vi "demo_Comparison Reports from CLI.vi"(11 "Stop Demo":refnum<user-event>) -> ()   [LabVIEW 2020]
panel:
  # "LabVIEW 2025 Q3 Beta - Comparison Reports from LabVIEW CLI\n\nThe LabVIEW CLI now includes the CreateComparisonReport operation which will generate VI Comparison reports. You can specify a report type of HTML, HTML (Single File), Microsoft Word, Plain Text, or XML.\n\nLearn more about the LabVIEW 2025 Q3 Beta program at https://www.ni.com/beta."
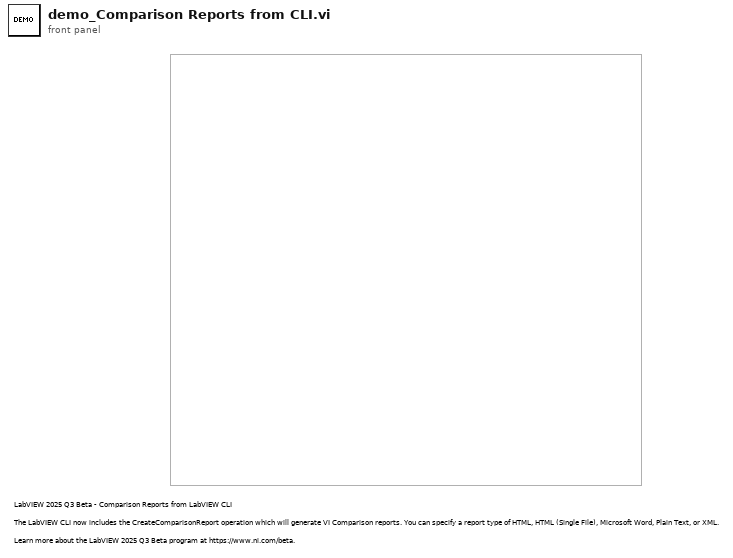
[diagram p1: front panel]
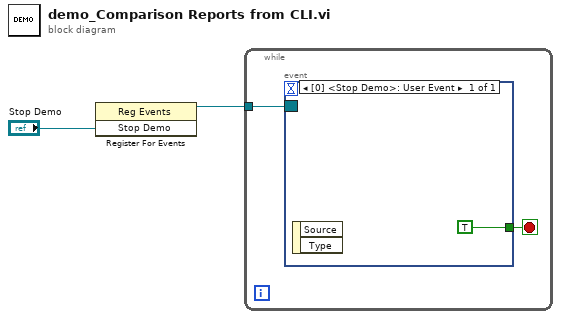
[diagram p0: block diagram]
diagram:
  n1 = register-events("Stop Demo") -> (reference out=w1:refnum<event-registration>)  [unwired: 2 in, 1 out]
  n2 = while {
    tunnel: w1 -> [w4]
    stop <- w3 stop-if-true
    n3 = event shown="[0] <Stop Demo>: User Event" {
      selector: w4 -> [_]
      dyn-events: _ -> [_]
      timeout: _ -> [_]
      tunnel: [TRUE] -> w3
      event User Event {
        n4 = event-data() -> ()  [unwired: 1 in, 2 out]
      }
    }
  }
